vi "ModelSimulationAdv.vi"() -> ()   [LabVIEW 2015]
uses:
  Classes/CAlex2/TypeDef/LowerBodyDim.ctl
  Classes/ForceField/TypeDef/FF_Gains.ctl
  Classes/CAlex2/CAlex2.lvclass
  Classes/CAlex2-Display/CAlex2_Display.lvclass
  Classes/ForceField/ForceField.lvclass
  <vilib>/Platform/TimedLoop/XDataNode/timing_clust.ctl
  <vilib>/Platform/TimedLoop/XDataNode/nitl_modes.ctl
  <vilib>/Platform/TimedLoop/XDataNode/wakeup.ctl
  Classes/ForceField/FF_SetGains.vi
  <vilib>/Analysis/BLAS.llb/dgemv - General Matrix-Vector Product (DBL).vi
  <vilib>/Platform/TimedLoop/XDataNode/XDataNode.xnode
  <vilib>/Platform/TimedLoop/XDataNode/XDNodeRunTimeDep.lvlib
  Classes/SerialChain-Cable/SerialChain-Cable.lvclass
  <vilib>/Analysis/NI_AALBLAS.lvlib
  <vilib>/ptbypt/NI_PtbyPt.lvlib
panel:
  in  "ExtraWeight(kg)":cluster{"Thigh":dbl, "Shank":dbl}
  out "Array":dbl[](array[numeric])
  out "AverageTraj":dbl[][](array[numeric])
  out "Joint Angles 3":dbl(graph)
  out "Ankle Location":T1(graph)
  in  "ForceField":enum16{"Old", "Adv"}(ring)
  out "size(s)":i32[](array[numeric])
  in  "stop":bool
  in  "Speed":dbl(slide) scale=0.1..1.0
  out "Iteration Duration":i64
  out "Joint Angles":T2(graph)
  in  "Reset":bool
  in  "Play":bool
  out "Joint Angles":dbl[][](graph)
  out "AnkleTraj dup":dbl[][](array[numeric])=[[0.37183265375099783, -0.7753745975904054, 0.0], [0.37289482382685957, -0.7748969789550374, 0.0], [0.373493623426573, -0.774628944735343, 0.0], [0.37411977937897245, -0.7743495847216937, 0.0], [0.37433541633017775, -0.7742546779467274, 0.0], [0.37425855125757534, -0.7742906050038265, 0.0], [0.37384605819479033, -0.774472841116272, 0.0], [0.37296121505608076, -0.7748580324475733, 0.0], [0.37170692962948126, -0.7753928087899727, 0.0], [0.3700602785380804, -0.7760822332687248, 0.0], [0.36809143852899284, -0.7768866046659747, 0.0], [0.36568836065849897, -0.7778423221117037, 0.0], [0.36313552913237124, -0.7788278813089, 0.0], [0.3601118692047611, -0.7799584423849573, 0.0], [0.3572321518028252, -0.7809989203616594, 0.0], [0.35378972494099115, -0.7822011715240718, 0.0], [0.35059287638745984, -0.7832774768890238, 0.0], [0.3467578061484453, -0.7845221886070235, 0.0], [0.3432982823348635, -0.7856008298535131, 0.0], [0.33934836631794885, -0.7867910445374475, 0.0], [0.33541324452244614, -0.7879258693076385, 0.0], [0.3314474700295142, -0.789029178751681, 0.0], [0.32715884390484884, -0.7901684748000672, 0.0], [0.3231117563662566, -0.7912012543919054, 0.0], [0.3184724786883741, -0.7923291759292822, 0.0], [0.314162029124302, -0.7933285258974756, 0.0], [0.3094336910282637, -0.7943728574273302, 0.0], [0.3048815845425384, -0.7953276067807286, 0.0], [0.30006249829487697, -0.7962839160327793, 0.0], [0.2952110578635034, -0.797190712968026, 0.0], [0.2903579578045672, -0.7980471058277165, 0.0], [0.2853196096836144, -0.7988732306589323, 0.0], [0.28033113007614985, -0.7996408813366376, 0.0], [0.2749999968937097, -0.8003945622659994, 0.0], [0.27005660632103534, -0.801037842898324, 0.0], [0.26454255052510184, -0.8016912636825307, 0.0], [0.2594436259092606, -0.8022365009693144, 0.0], [0.25384070753157423, -0.8027682840071089, 0.0], [0.24872618036880667, -0.8031916470946026, 0.0], [0.2431628291886645, -0.8035855761699472, 0.0], [0.237850957225839, -0.8038946687980629, 0.0], [0.23220014909346698, -0.8041535831823374, 0.0], [0.22702101700957686, -0.8043243026289639, 0.0], [0.22132859036727104, -0.8044455086499704, 0.0], [0.2161303736065503, -0.8044862796442338, 0.0], [0.21053389057023572, -0.8044652948207722, 0.0], [0.20494606247739322, -0.8043670725575002, 0.0], [0.1996795642462802, -0.804209365734722, 0.0], [0.19387414206660697, -0.803959487604845, 0.0], [0.18860569655152407, -0.8036662143242687, 0.0], [0.18290985424210632, -0.8032746472778416, 0.0], [0.17763852673112943, -0.80284451181639, 0.0], [0.1720637346201731, -0.8023168832402672, 0.0], [0.16670541014624216, -0.8017411231307242, 0.0], [0.16124688034804877, -0.8010855122017577, 0.0], [0.1559100209598843, -0.800376945216661, 0.0], [0.15027133848749125, -0.7995524032540577, 0.0], [0.14506338428592272, -0.7987270788629399, 0.0], [0.13937552048376003, -0.797759709715296, 0.0], [0.134221407365669, -0.7968187612931736, 0.0], [0.12856350148196946, -0.7957309833621973, 0.0], [0.12328836974914918, -0.7946723721393905, 0.0], [0.11749057966524709, -0.7934558221054675, 0.0], [0.11228354529372929, -0.79232840321483, 0.0], [0.10644084465997686, -0.7910119517196016, 0.0], [0.10095291735243607, -0.7897521646217016, 0.0], [0.0949742465260796, -0.7883287460106716, 0.0], [0.08932119053218368, -0.7869521967616934, 0.0], [0.08343964132641435, -0.785483040113578, 0.0], [0.07762692966656667, -0.7839991497744392, 0.0], [0.07135683936790438, -0.7823613070633205, 0.0], [0.0656352421659741, -0.7808325842640069, 0.0], [0.05928812168117539, -0.7791024245187889, 0.0], [0.05326784691840181, -0.7774341704120975, 0.0], [0.04720152296919525, -0.7757070205082308, 0.0], [0.04113274195842884, -0.7739569091825252, 0.0], [0.035073495589465875, -0.7721639239188988, 0.0], [0.029092778510038497, -0.7703645301795483, 0.0], [0.023148090702767327, -0.7685386619074226, 0.0], [0.01733760024588965, -0.7667249115039706, 0.0], [0.011116829949580742, -0.7647479503952259, 0.0], [0.005295634045588998, -0.7628511751120268, 0.0], [-0.00043876377786242204, -0.7609635946087108, 0.0], [-0.006342201549036891, -0.7589715759608368, 0.0], [-0.011929098616239558, -0.7570671623466152, 0.0], [-0.01774704906579269, -0.7550426162385022, 0.0], [-0.023541544919570417, -0.7530086819325862, 0.0], [-0.028957258939425468, -0.7510705734835252, 0.0], [-0.034698138313621396, -0.7490009106985951, 0.0], [-0.04008729757012036, -0.7470392767080659, 0.0], [-0.04574900793341244, -0.7449658783801192, 0.0], [-0.051320828424748444, -0.7429059583063504, 0.0], [-0.05677467622680521, -0.7408648077406232, 0.0], [-0.06226454675363144, -0.7388113211597775, 0.0], [-0.0676389204429593, -0.7367811542598004, 0.0], [-0.0728442278462823, -0.7348053465420634, 0.0], [-0.0782357241582145, -0.7327620142872742, 0.0], [-0.0836394929256932, -0.7306888915502054, 0.0], [-0.0887720530740976, -0.7287105862736893, 0.0], [-0.09389454917760404, -0.726732998735621, 0.0], [-0.09886685610474269, -0.7247987455299281, 0.0], [-0.10383869318508343, -0.722867469607505, 0.0], [-0.10852151332262627, -0.7210522484792419, 0.0], [-0.113409207857913, -0.7191438167829669, 0.0], [-0.11793809256479892, -0.7173929476150898, 0.0], [-0.12254124998410773, -0.7155942737218733, 0.0], [-0.12693686993795159, -0.7139135811901516, 0.0], [-0.13161630521760578, -0.7121241599601726, 0.0], [-0.13581258018488523, -0.7105322342176328, 0.0], [-0.14027599616508363, -0.708881590455069, 0.0], [-0.14450030181936724, -0.7073181803603608, 0.0], [-0.14877060013956167, -0.7057871374866982, 0.0], [-0.1529901004972806, -0.7042851345154005, 0.0], [-0.15718019582987636, -0.7028327254328446, 0.0], [-0.16122244521688234, -0.7014823298049171, 0.0], [-0.1653162445977395, -0.7001418829804374, 0.0], [-0.16929374726325766, -0.69889983696989, 0.0], [-0.1734783601455121, -0.6976299042507634, 0.0], [-0.1770966735528886, -0.6965984300714734, 0.0], [-0.18114059602104032, -0.6955090442952979, 0.0], [-0.184935925009572, -0.6945583547855383, 0.0], [-0.18878423624534665, -0.6937178759316448, 0.0], [-0.19242257225482037, -0.6929866662389191, 0.0], [-0.19615973677621426, -0.6923787119922514, 0.0], [-0.19978175605815884, -0.6919052431255679, 0.0], [-0.20337246600553527, -0.6915188855358476, 0.0], [-0.20682426326370662, -0.6913009470371396, 0.0], [-0.2102769928693155, -0.6912104861499663, 0.0], [-0.2136766885217551, -0.6912634393978416, 0.0], [-0.21702450391347713, -0.6914592765636891, 0.0], [-0.22023476858846222, -0.6917523077549168, 0.0], [-0.22331956369937084, -0.6922362445610458, 0.0], [-0.22636686575938247, -0.6928341134395831, 0.0], [-0.22922823266369957, -0.693665641519721, 0.0], [-0.23192753904420305, -0.6945320687978396, 0.0], [-0.23441321506243118, -0.6956651784863382, 0.0], [-0.2368821322965693, -0.696925825030893, 0.0], [-0.2389547948215033, -0.6982781184291174, 0.0], [-0.24110089510899507, -0.6998876962445497, 0.0], [-0.24287465696440025, -0.7014423387913367, 0.0], [-0.2446742043707928, -0.7033559882647625, 0.0], [-0.24620697206049796, -0.7051112811196629, 0.0], [-0.24764820933713433, -0.7071011257159412, 0.0], [-0.2490230174457068, -0.7091334575948564, 0.0], [-0.25031144941568106, -0.7112798262977702, 0.0], [-0.2514427644386446, -0.7134317431304611, 0.0], [-0.2524929750018052, -0.7155589393861124, 0.0], [-0.25350072515651867, -0.7178246947777653, 0.0], [-0.254380221322995, -0.719927018561745, 0.0], [-0.2552616792998671, -0.722267545511442, 0.0], [-0.2560251567346829, -0.7243835323272311, 0.0], [-0.25680867032020616, -0.726693828115996, 0.0], [-0.2575062201163926, -0.7288676957769442, 0.0], [-0.25816974272182763, -0.7310791287719528, 0.0], [-0.2588252699568618, -0.7333147576395038, 0.0], [-0.25942071073535394, -0.7354274902405354, 0.0], [-0.26003385044795635, -0.7376236111250145, 0.0], [-0.26059715988663323, -0.7396714097897619, 0.0], [-0.2612200470159218, -0.7418991707604716, 0.0], [-0.2617377263415781, -0.7437515197313708, 0.0], [-0.2623744155157041, -0.7459309017913354, 0.0], [-0.26297860529215933, -0.7479575530548156, 0.0], [-0.26358132537438494, -0.7499323028969112, 0.0], [-0.26418697767727833, -0.7518509648059314, 0.0], [-0.264777188672622, -0.7536804383160631, 0.0], [-0.2654198112780903, -0.7556471666562012, 0.0], [-0.2660113415426726, -0.7574533877863839, 0.0], [-0.26659672532042766, -0.7592299713856276, 0.0], [-0.26721269508289713, -0.7611377923270144, 0.0], [-0.2677374078136171, -0.7627913062390148, 0.0], [-0.2683173793927711, -0.7646159197743312, 0.0], [-0.2688101626362109, -0.7661970294615574, 0.0], [-0.26934819761677037, -0.7679265486285046, 0.0], [-0.26984717901082056, -0.7695254496619343, 0.0], [-0.2703347490737253, -0.7711106818083092, 0.0], [-0.27080781288628913, -0.772685255158352, 0.0], [-0.2712845477065148, -0.7742376677421277, 0.0], [-0.27172652145721626, -0.7757296853818727, 0.0], [-0.2721619027572711, -0.7772206684253814, 0.0], [-0.2725457806411501, -0.7786164445559429, 0.0], [-0.27292845491681295, -0.7800794437434274, 0.0], [-0.27325630885853164, -0.7814606263774184, 0.0], [-0.27356303285043426, -0.7828369241522507, 0.0], [-0.2738096548030798, -0.7841627795610804, 0.0], [-0.27402878883574844, -0.7854881888275353, 0.0], [-0.274186228925163, -0.7867626824220673, 0.0], [-0.2743073583286294, -0.7880418506185414, 0.0], [-0.27438738928150447, -0.7892385417358527, 0.0], [-0.2744288342261834, -0.7904689488865955, 0.0], [-0.27441035565444816, -0.7916168524596761, 0.0], [-0.2743634125063062, -0.7927596786734321, 0.0], [-0.2742574236518008, -0.7938718639614482, 0.0], [-0.2741374078183783, -0.7949318812614583, 0.0], [-0.27393887109827364, -0.7960858921110872, 0.0], [-0.2737038263626721, -0.7970832634677752, 0.0], [-0.27341166537655365, -0.798171028508889, 0.0], [-0.2730650444966486, -0.7991339477482047, 0.0], [-0.2726347689249194, -0.8001615272613687, 0.0], [-0.2721534360578481, -0.8011109416356981, 0.0], [-0.27152846952377346, -0.8021552451662262, 0.0], [-0.2708770070319027, -0.8030965774960956, 0.0], [-0.2700172155863569, -0.8041445311604927, 0.0], [-0.26913106108347484, -0.805109858166045, 0.0], [-0.2680068487918412, -0.8061885367916513, 0.0], [-0.2668211514937952, -0.8072184001367346, 0.0], [-0.2654878391152534, -0.8082713109319719, 0.0], [-0.2640317937400684, -0.8093315890960024, 0.0], [-0.26237379458714477, -0.8104381846073867, 0.0], [-0.26068727382666523, -0.8115060789128818, 0.0], [-0.2587495769707093, -0.8126439793150716, 0.0], [-0.25671166521781325, -0.8137870428806746, 0.0], [-0.2546156310828552, -0.8148983667177427, 0.0], [-0.2522381549641083, -0.8161021500951877, 0.0], [-0.2499761368107293, -0.8171988530971919, 0.0], [-0.2474711463082518, -0.8183702224831575, 0.0], [-0.2450060689856413, -0.8194795582043639, 0.0], [-0.24244470949827496, -0.8205997730249799, 0.0], [-0.23993477307897781, -0.821661641193336, 0.0], [-0.2373917701683875, -0.8227104193851609, 0.0], [-0.23480473958874443, -0.8237435592023392, 0.0], [-0.23221757387585168, -0.8247537872359236, 0.0], [-0.22965895358119026, -0.8257246471199526, 0.0], [-0.22711604521835227, -0.8266670541451011, 0.0], [-0.22467194478881602, -0.8275515105824701, 0.0], [-0.2222209361099186, -0.828418398645937, 0.0], [-0.21975095200379302, -0.8292715405676382, 0.0], [-0.21740179408864782, -0.8300646562631699, 0.0], [-0.2150218549152477, -0.8308488450960334, 0.0], [-0.21269276783515087, -0.8316005563577531, 0.0], [-0.2105430277629809, -0.8322800833587969, 0.0], [-0.20827546261146768, -0.8329810666985676, 0.0], [-0.20616611188279502, -0.8336227899995121, 0.0], [-0.20411247571039182, -0.8342342912086944, 0.0], [-0.2019978531568194, -0.8348527927379376, 0.0], [-0.20015106125248622, -0.835383430255904, 0.0], [-0.19815292207435609, -0.8359473626823527, 0.0], [-0.19645607999172088, -0.8364189829271711, 0.0], [-0.19464053492952343, -0.8369158132866583, 0.0], [-0.19307405926458887, -0.837338306633453, 0.0], [-0.19139803881526166, -0.8377833938319692, 0.0], [-0.18962018754632556, -0.8382482281998148, 0.0], [-0.18824260076912852, -0.8386033398660642, 0.0], [-0.1867633360321964, -0.8389793558486134, 0.0], [-0.18547833013150733, -0.8393014955259506, 0.0], [-0.18404141743744645, -0.8396562208809251, 0.0], [-0.18278247041905893, -0.8399627646858725, 0.0], [-0.18140807652754443, -0.8402927271900011, 0.0], [-0.18012494884891897, -0.8405961811142164, 0.0], [-0.1788289309698709, -0.8408988399639594, 0.0], [-0.17747462776908626, -0.8412099050582688, 0.0], [-0.17619382108109571, -0.8415005768042629, 0.0], [-0.17481346130734696, -0.8418093850591277, 0.0], [-0.17340829015016793, -0.8421196068543741, 0.0], [-0.1719694132738892, -0.842432616487675, 0.0], [-0.17047884539720298, -0.8427527384267661, 0.0], [-0.16896770404045502, -0.843072807600878, 0.0], [-0.1673780501531782, -0.84340478181457, 0.0], [-0.16571906452660776, -0.8437464035465461, 0.0], [-0.16404147499149918, -0.8440869618649394, 0.0], [-0.16228213634532412, -0.8444392151349265, 0.0], [-0.16047364442066228, -0.8447957743706607, 0.0], [-0.1586514507170836, -0.8451499896818444, 0.0], [-0.15677822979604894, -0.8455086788850721, 0.0], [-0.15483004182304438, -0.8458762665312334, 0.0], [-0.15283113439288662, -0.8462475387577932, 0.0], [-0.15072388689399357, -0.8466328389003069, 0.0], [-0.14872295822956122, -0.8469927691964696, 0.0], [-0.14650702271158547, -0.847385139741527, 0.0], [-0.14442166132674084, -0.8477481694081889, 0.0], [-0.1422666720786283, -0.8481172868947848, 0.0], [-0.14004673814526042, -0.8484910648578541, 0.0], [-0.13796406790621085, -0.8488358398219539, 0.0], [-0.13572869301500584, -0.8491996022657746, 0.0], [-0.13358391000669767, -0.8495425544447857, 0.0], [-0.13140858934261096, -0.8498843882979255, 0.0], [-0.12928110336475632, -0.8502129140790096, 0.0], [-0.12704531611413403, -0.8505519396803537, 0.0], [-0.12499877452630204, -0.8508567808565243, 0.0], [-0.12287895472414473, -0.8511669920612306, 0.0], [-0.1209871435845552, -0.8514391483290421, 0.0], [-0.11891710432316879, -0.8517318300467451, 0.0], [-0.11706935003037391, -0.8519886162558002, 0.0], [-0.11522229341616635, -0.8522411020733642, 0.0], [-0.11351709372269617, -0.8524704787231319, 0.0], [-0.11174322345590623, -0.8527053249622711, 0.0], [-0.11013622737131207, -0.8529147618458993, 0.0], [-0.10840840557341808, -0.8531364414159233, 0.0], [-0.10701529650561606, -0.8533125360256351, 0.0], [-0.10536501640381091, -0.8535181014042106, 0.0], [-0.10383529190748454, -0.8537057161586962, 0.0], [-0.10238143017378959, -0.8538814096088274, 0.0], [-0.10082932866972373, -0.854066181686951, 0.0], [-0.09936778885974791, -0.8542375272359429, 0.0], [-0.09782548082175646, -0.8544155765474297, 0.0], [-0.0963157931390409, -0.8545871110310665, 0.0], [-0.09474769022157203, -0.854762396513045, 0.0], [-0.09318198152710554, -0.8549345022846709, 0.0], [-0.09154856137331283, -0.8551109351178154, 0.0], [-0.08990834228076758, -0.8552849215694632, 0.0], [-0.088198444687737, -0.8554628953887149, 0.0], [-0.08648663207162453, -0.8556376015115305, 0.0], [-0.08468618696227526, -0.8558175989984749, 0.0], [-0.08287167596264519, -0.8559951191779169, 0.0], [-0.08097949268135497, -0.8561760880823152, 0.0], [-0.07903148956315978, -0.8563579629636042, 0.0], [-0.07704161240048532, -0.8565391221986036, 0.0], [-0.07502566632690028, -0.8567178812545901, 0.0], [-0.07282142574034856, -0.8569078409138489, 0.0], [-0.07076608151912692, -0.8570798219419018, 0.0], [-0.06835711622559534, -0.8572750411585485, 0.0], [-0.06613254008617091, -0.8574492739066633, 0.0], [-0.06355061805798805, -0.8576441765080185, 0.0], [-0.06106420248426459, -0.8578244406207083, 0.0], [-0.05850268624516532, -0.8580025935368184, 0.0], [-0.055736260696897, -0.8581862830569933, 0.0], [-0.05305406859854181, -0.8583558796759434, 0.0], [-0.050262421932745986, -0.8585233303202323, 0.0], [-0.04736702971716894, -0.8586874080081011, 0.0], [-0.044370286732769645, -0.8588467922743324, 0.0], [-0.041531306378691873, -0.858988078838129, 0.0], [-0.03839991406525789, -0.8591328669596852, 0.0], [-0.03510860090786879, -0.8592725569099622, 0.0], [-0.03210990117282504, -0.8593887569585896, 0.0], [-0.028899478532724704, -0.8595012427721156, 0.0], [-0.025823678520056043, -0.8595976180772692, 0.0], [-0.022617832756158897, -0.859685893536088, 0.0], [-0.01946792858750787, -0.8597607865717275, 0.0], [-0.016388976031073983, -0.8598223381851606, 0.0], [-0.013167726108472215, -0.8598744713081619, 0.0], [-0.010251216509382356, -0.8599107816034928, 0.0], [-0.007019606669465612, -0.8599386941101604, 0.0], [-0.004153763070109593, -0.8599528219186598, 0.0], [-0.0010910884263649967, -0.859956271256102, 0.0], [0.001778124897785133, -0.8599488154199191, 0.0], [0.004647360708474891, -0.8599306751781897, 0.0], [0.007474672404238891, -0.8599024106472315, 0.0], [0.010355664289539997, -0.8598628527522061, 0.0], [0.013069752444236783, -0.8598149395701302, 0.0], [0.01565097819637608, -0.8597608617255861, 0.0], [0.018464189530154194, -0.8596909628742213, 0.0], [0.020971142300671836, -0.8596199682875074, 0.0], [0.02373313451673249, -0.8595314661119279, 0.0], [0.026241847162740032, -0.859442077835348, 0.0], [0.02896355621561992, -0.8593351658357784, 0.0], [0.031561304479187265, -0.8592236525940238, 0.0], [0.03421311230968467, -0.8591002220711204, 0.0], [0.03692509235563076, -0.8589642546371237, 0.0], [0.03966199276671022, -0.8588161876750965, 0.0], [0.04233321473653107, -0.8586615454189499, 0.0], [0.04500898398863215, -0.8584958883725464, 0.0], [0.04774489004844869, -0.8583155343357147, 0.0], [0.05036852727515613, -0.8581319745907592, 0.0], [0.05317339321487827, -0.8579249192964813, 0.0], [0.055798644180901726, -0.8577203942779614, 0.0], [0.05851843148614406, -0.8574972766947069, 0.0], [0.06122614212627327, -0.8572652071642932, 0.0], [0.0640107179210352, -0.8570141205377868, 0.0], [0.066691883462811, -0.8567630906049144, 0.0], [0.06954690889383948, -0.8564847261034455, 0.0], [0.07222822506589574, -0.8562138180184402, 0.0], [0.07542250396384256, -0.8558816792851693, 0.0], [0.0781719810318635, -0.8555841106898108, 0.0], [0.08139890251569763, -0.8552270930677746, 0.0], [0.08450389791313062, -0.8548725915629658, 0.0], [0.08773326273118319, -0.8544901441486166, 0.0], [0.09090642645414464, -0.854104783508446, 0.0], [0.09423999387967696, -0.8536883980846051, 0.0], [0.09750187723856218, -0.8532660006092561, 0.0], [0.1009018177825952, -0.8528153371744314, 0.0], [0.1041666709264735, -0.8523687507035258, 0.0], [0.10761630667780497, -0.8518868915180231, 0.0], [0.11074845594993368, -0.8514315701081683, 0.0], [0.11421463157333586, -0.8509189161811136, 0.0], [0.11738828663298527, -0.8504348099207938, 0.0], [0.12061003539211371, -0.8499339763267597, 0.0], [0.12377847214797102, -0.8494281235205758, 0.0], [0.12708458841920295, -0.8488895628043887, 0.0], [0.13016688827131792, -0.848375207862568, 0.0], [0.1333610916696111, -0.8478330249247403, 0.0], [0.13647626865151896, -0.8472928272446203, 0.0], [0.1396480343049928, -0.8467332182857404, 0.0], [0.14274536276537236, -0.8461742791491627, 0.0], [0.14598771932507743, -0.845581902804462, 0.0], [0.14890986227024136, -0.8450377521723433, 0.0], [0.1522270134213003, -0.8444105384630858, 0.0], [0.15532553945701422, -0.8438148464185712, 0.0], [0.15845498938830296, -0.8432043069254598, 0.0], [0.1614889015454986, -0.8426028519161191, 0.0], [0.1645666116878986, -0.841982843672705, 0.0], [0.1675741369540738, -0.8413686429892312, 0.0], [0.17046967399268204, -0.8407689299249975, 0.0], [0.17340469189720858, -0.8401536828041312, 0.0], [0.17612716517541172, -0.8395760151571943, 0.0], [0.17892301069413136, -0.8389753104777607, 0.0], [0.18165778429941154, -0.838381186768423, 0.0], [0.18415151787095663, -0.8378335332382447, 0.0], [0.18669339618022673, -0.8372717339545527, 0.0], [0.18905363464157615, -0.8367432081061068, 0.0], [0.19135324597196007, -0.8362278102306224, 0.0], [0.19363888485475977, -0.835709303566087, 0.0], [0.19590158290764315, -0.8351967462825411, 0.0], [0.1981084640038252, -0.8346931100438553, 0.0], [0.20033022729261885, -0.83418524884933, 0.0], [0.20259605689944776, -0.833665550948625, 0.0], [0.204901890440473, -0.8331324000017677, 0.0], [0.2073263385550317, -0.832570336107055, 0.0], [0.20979040241561736, -0.8319946891819853, 0.0], [0.21248896162809622, -0.8313596057342136, 0.0], [0.2150565630550852, -0.830750022361683, 0.0], [0.2179907905266466, -0.8300447061782359, 0.0], [0.22079792544536309, -0.8293630186961082, 0.0], [0.22378446417723674, -0.828627414972503, 0.0], [0.2267101506860001, -0.8278975003771158, 0.0], [0.22993841717261024, -0.8270787890188973, 0.0], [0.23296514070884217, -0.8263008813606285, 0.0], [0.23615343240265585, -0.825468032758038, 0.0], [0.23921892931773792, -0.824654146994607, 0.0], [0.24252743094243195, -0.8237622193619464, 0.0], [0.24557349850440333, -0.822927335774595, 0.0], [0.24877572680170718, -0.8220370922257707, 0.0], [0.2517901425415419, -0.8211837168887886, 0.0], [0.2550128597037762, -0.8202592598352787, 0.0], [0.2578981453454072, -0.8194170964491038, 0.0], [0.2610146145836939, -0.8184957785318425, 0.0], [0.26388548653260374, -0.8176323515222093, 0.0], [0.26675057068370417, -0.8167598230099201, 0.0], [0.2695178402960374, -0.8159053242860688, 0.0], [0.27232531831880064, -0.8150257302621371, 0.0], [0.2749435624610046, -0.8141965433092677, 0.0], [0.27769696793626447, -0.8133118176593679, 0.0], [0.2802063212271111, -0.8124965604428448, 0.0], [0.28285269700734705, -0.8116261291001333, 0.0], [0.2853681052357947, -0.8107887997983884, 0.0], [0.2879112490380726, -0.8099321466933329, 0.0], [0.29039526587283787, -0.8090850305927854, 0.0], [0.29276494026480815, -0.8082681838187457, 0.0], [0.2952725006554657, -0.8073934026365, 0.0], [0.29755405702431903, -0.8065889536156597, 0.0], [0.30000649001559, -0.8057148373344248, 0.0], [0.30223738185111115, -0.8049108096460895, 0.0], [0.3046260290344815, -0.8040405201512473, 0.0], [0.3067465864499216, -0.8032598902083721, 0.0], [0.30900254170215785, -0.802421524563772, 0.0], [0.31098481023502517, -0.801677341465603, 0.0], [0.31308613919629935, -0.8008815451475904, 0.0], [0.31489460499025823, -0.8001904675097968, 0.0], [0.31681506677079885, -0.7994505313042297, 0.0], [0.318505013060268, -0.7987939467899835, 0.0], [0.3203037190245617, -0.7980890086554995, 0.0], [0.3219528440359778, -0.797437071431937, 0.0], [0.32366911018666833, -0.7967521646516664, 0.0], [0.3254216921724232, -0.7960458041553538, 0.0], [0.32712704621727495, -0.795351518173878, 0.0], [0.3290293092012364, -0.7945688036216725, 0.0], [0.3308473666700556, -0.7938127295055969, 0.0], [0.33296376759017093, -0.7929229766820975, 0.0], [0.334932220404212, -0.7920863292322609, 0.0], [0.337180395170873, -0.7911206162524718, 0.0], [0.33935673859080817, -0.7901757239041011, 0.0], [0.34163736031660535, -0.78917503855842, 0.0], [0.34403234844406066, -0.7881136551471178, 0.0], [0.3461839921685177, -0.7871504177049249, 0.0], [0.3486115004743213, -0.7860538836945515, 0.0], [0.35060255233506765, -0.7851460399823808, 0.0], [0.3527788851356809, -0.7841473112638164, 0.0], [0.3545976299933107, -0.783306390513216, 0.0], [0.3564533527366056, -0.7824443739675445, 0.0], [0.35805011929249386, -0.7816995677937202, 0.0], [0.3595694107302563, -0.7809884623637544, 0.0], [0.36091162353209566, -0.7803607510769153, 0.0], [0.36214910788724897, -0.7797817215270448, 0.0], [0.36333794462930863, -0.7792279294893029, 0.0], [0.36447171537128087, -0.778702413584851, 0.0], [0.3654410245748628, -0.7782563066425645, 0.0], [0.36657730897196084, -0.777737299247806, 0.0], [0.36742052655401913, -0.7773538478430514, 0.0], [0.36858563173190617, -0.7768266280103568, 0.0], [0.36942057890451696, -0.7764499087497039, 0.0], [0.37061429689154934, -0.7759115502341369, 0.0], [0.3714117663491737, -0.7755523212160451, 0.0]]
  in  "Relative Weight":dbl[](array[numeric]) format="%#.3f"
  out "ActualTorque":dbl[](array[numeric]) format="%#.6f"
  in  "Gains":T3
  out "FieldForce":dbl[](array[numeric])
  in  "InitDisplay":bool
  out "ActiveTraj":dbl[][](array[numeric])
  in  "BodyWtComp?(F)":bool
  in  "CuffWtComp?(F)":bool=TRUE
  in  "InitFF":bool
  in  "Weight(1e-6)":dbl=1e-06 format="%#_13g"
  in  "LegProperties":T4={"BodyDim(m)"={"ThighLt"=0.42, "ShankLt"=0.42, "HipWd"=0.32}, "BodyWt(kg)"={"Thigh"=0.0, "Shank"=0.0}, "CuffLoc(m)"={"HipCuffWd"=0.4, "HipCuffHt"=0.1, "HipCuffFwdShift"=0.0, "ThighCuffToKnee"=0.25, "ThighCuffDist"=0.04, "ShankCuffToKnee"=0.15}}
  out "FieldForceComp":dbl[](array[numeric]) format="%#.3f"
  out "ClosestPt":dbl[](array[numeric]) format="%#.3f"
  in  "TorqueError":T5
  in  "3D Curve":refnum<k7>(container)
  out "Torque Error":dbl[](array[numeric]) format="%#.3f"
  in  "QuadProg":enum16{"Tight", "Loose", "Adv"}(ring)
  out "Jacobian":dbl[][](array[numeric]) format="%#.4f"
  out "Joint Velocity (rad)":dbl[](array[numeric])
  out "Joint Angles (rad)":dbl[](array[numeric])
  out "DesiredTorque":dbl[](array[numeric]) format="%#.3f"
  in  "Update Arm":bool
  out "Iteration Duration 2":i64
  out "Ankle Position":dbl[](array[numeric]) format="%#.6f"
  out "Solved 2":bool
  out "Planned Tension":dbl[](array[numeric])
  in  "Joint Velocity (deg)":dbl[](array[numeric])=[0.0, 0.0, 0.0, 0.0]
  in  "Leg Joint Angles (deg)":dbl[](array[numeric])=[0.0, 0.0, 0.0, 0.0]
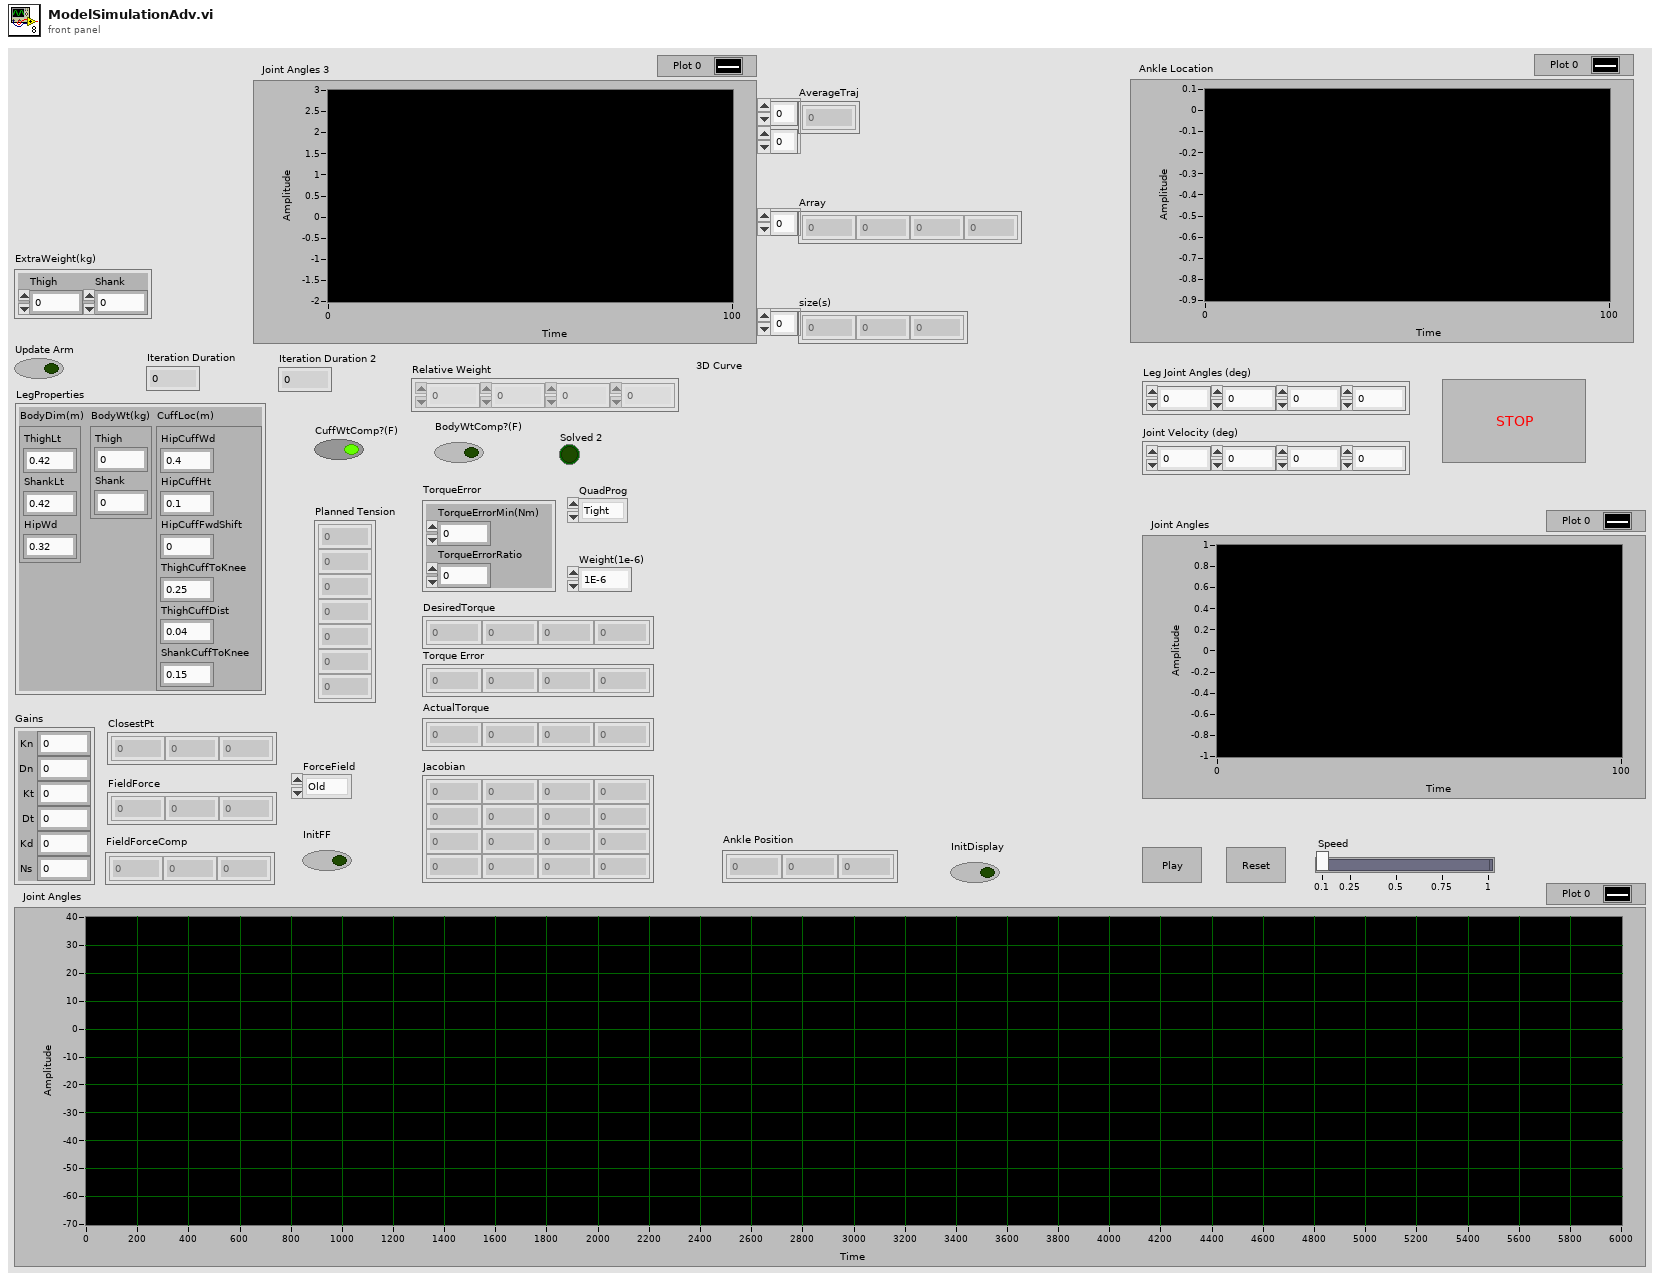
[diagram p1: front panel]
types:
  T1 = cluster{"EndEffInGCS[0]":dbl, "EndEffInGCS[1]":dbl, "EndEffInGCS[2]":dbl}
  T2 = cluster{"Leg Joint Angles (deg)[0]":dbl, "Leg Joint Angles (deg)[1]":dbl, "Leg Joint Angles (deg)[2]":dbl, "Leg Joint Angles (deg)[3]":dbl}
  T3 = typedef "ForceField.lvclass/FF_Gains.ctl" = cluster{"Kn":dbl, "Dn":dbl, "Kt":dbl, "Dt":dbl, "Kd":dbl, "Ns":dbl}
  T4 = typedef "CAlex2.lvclass/LowerBodyDim.ctl" = cluster{"BodyDim(m)":cluster{"ThighLt":dbl, "ShankLt":dbl, "HipWd":dbl}, "BodyWt(kg)":cluster{"Thigh":dbl, "Shank":dbl}, "CuffLoc(m)":cluster{"HipCuffWd":dbl, "HipCuffHt":dbl, "HipCuffFwdShift":dbl, "ThighCuffToKnee":dbl, "ThighCuffDist":dbl, "ShankCuffToKnee":dbl}}
  T5 = cluster{"TorqueErrorMin(Nm)":dbl, "TorqueErrorRatio":dbl}
  T6 = cluster{"Name":string, "Color":u32, "Style":i32, "Point Style":i32, "Name Visible":bool, "Allow Drag":bool, "Annotation Mode":i32, "Plot":i32, "Index":i32, "Position":cluster{"X":dbl, "Y":dbl}, "X Scale":u32, "Y Scale":u32, "Show Arrow":bool, "Lock Name":bool, "Plot Area":i32, "Label Offset":cluster{"X":dbl, "Y":dbl}}
  T7 = typedef "XDNodeRunTimeDep.lvlib/timing_clust.ctl" = cluster{"Expected End [f-1]":u64, "Actual End [f-1]":u64, "Finished Late? [f-1]":bool, "Expected End [i-1]":u64, "Actual End [i-1]":u64, "Finished Late? [i-1]":bool, "Expected Start [i]":u64, "Actual Start [i]":u64, "Expected Start [f]":u64, "Actual Start [f]":u64, "Source Name":string, "Structure Name":string, "Period":i64, "Deadline":i64, "Offset":i64, "Start":i64, "Priority":i32, "Timeout":i32, "Mode":T8, "Wakeup Reason":T9, "Error":errorcluster, "Source Type":string, "Secondary Source Type":string, "Global End Time":u64, "Global Start Time":u64, "Frame Duration":u64, "Iteration Duration":u64, "Assigned CPU":i32, "I/O Scan Engine Mode":u32}
  T8 = typedef "XDNodeRunTimeDep.lvlib/nitl_modes.ctl" = enum32{"No Change", "Process missed periods, maintain original phase", "Discard missed periods, maintain original phase", "Process missed periods, ignore original phase", "Discard missed periods, ignore original phase"}
  T9 = typedef "XDNodeRunTimeDep.lvlib/wakeup.ctl" = enum32{"Normal", "Aborted", "Asynchronous wakeup", "Timing source error", "Timed loop error", "Timeout"}
  T10 = cluster{"AxisLabel":string[], "AxisMax":dbl[], "AxisMin":dbl[]}
  T11 = typedef "SerialChain.lvclass/PointOnBody.ctl" = cluster{"Coord4":dbl[], "ID":i32}
  T12 = typedef "NI_Matrix.lvlib/RealMatrix.ctl" = dbl[][]
  T13 = cluster{"Name":string, "Color":u32, "Style":i32, "Point Style":i32, "Name Visible":bool, "Allow Drag":bool, "Annotation Mode":i32, "Plot":i32, "Index":i32, "Position":cluster{"X":dbl, "Y":dbl}, "X Scale":u32, "Y Scale":u32, "Show Arrow":bool, "Lock Name":bool, "Plot Area":i32, "Label Offset":cluster{"X":dbl, "Y":dbl}}[]
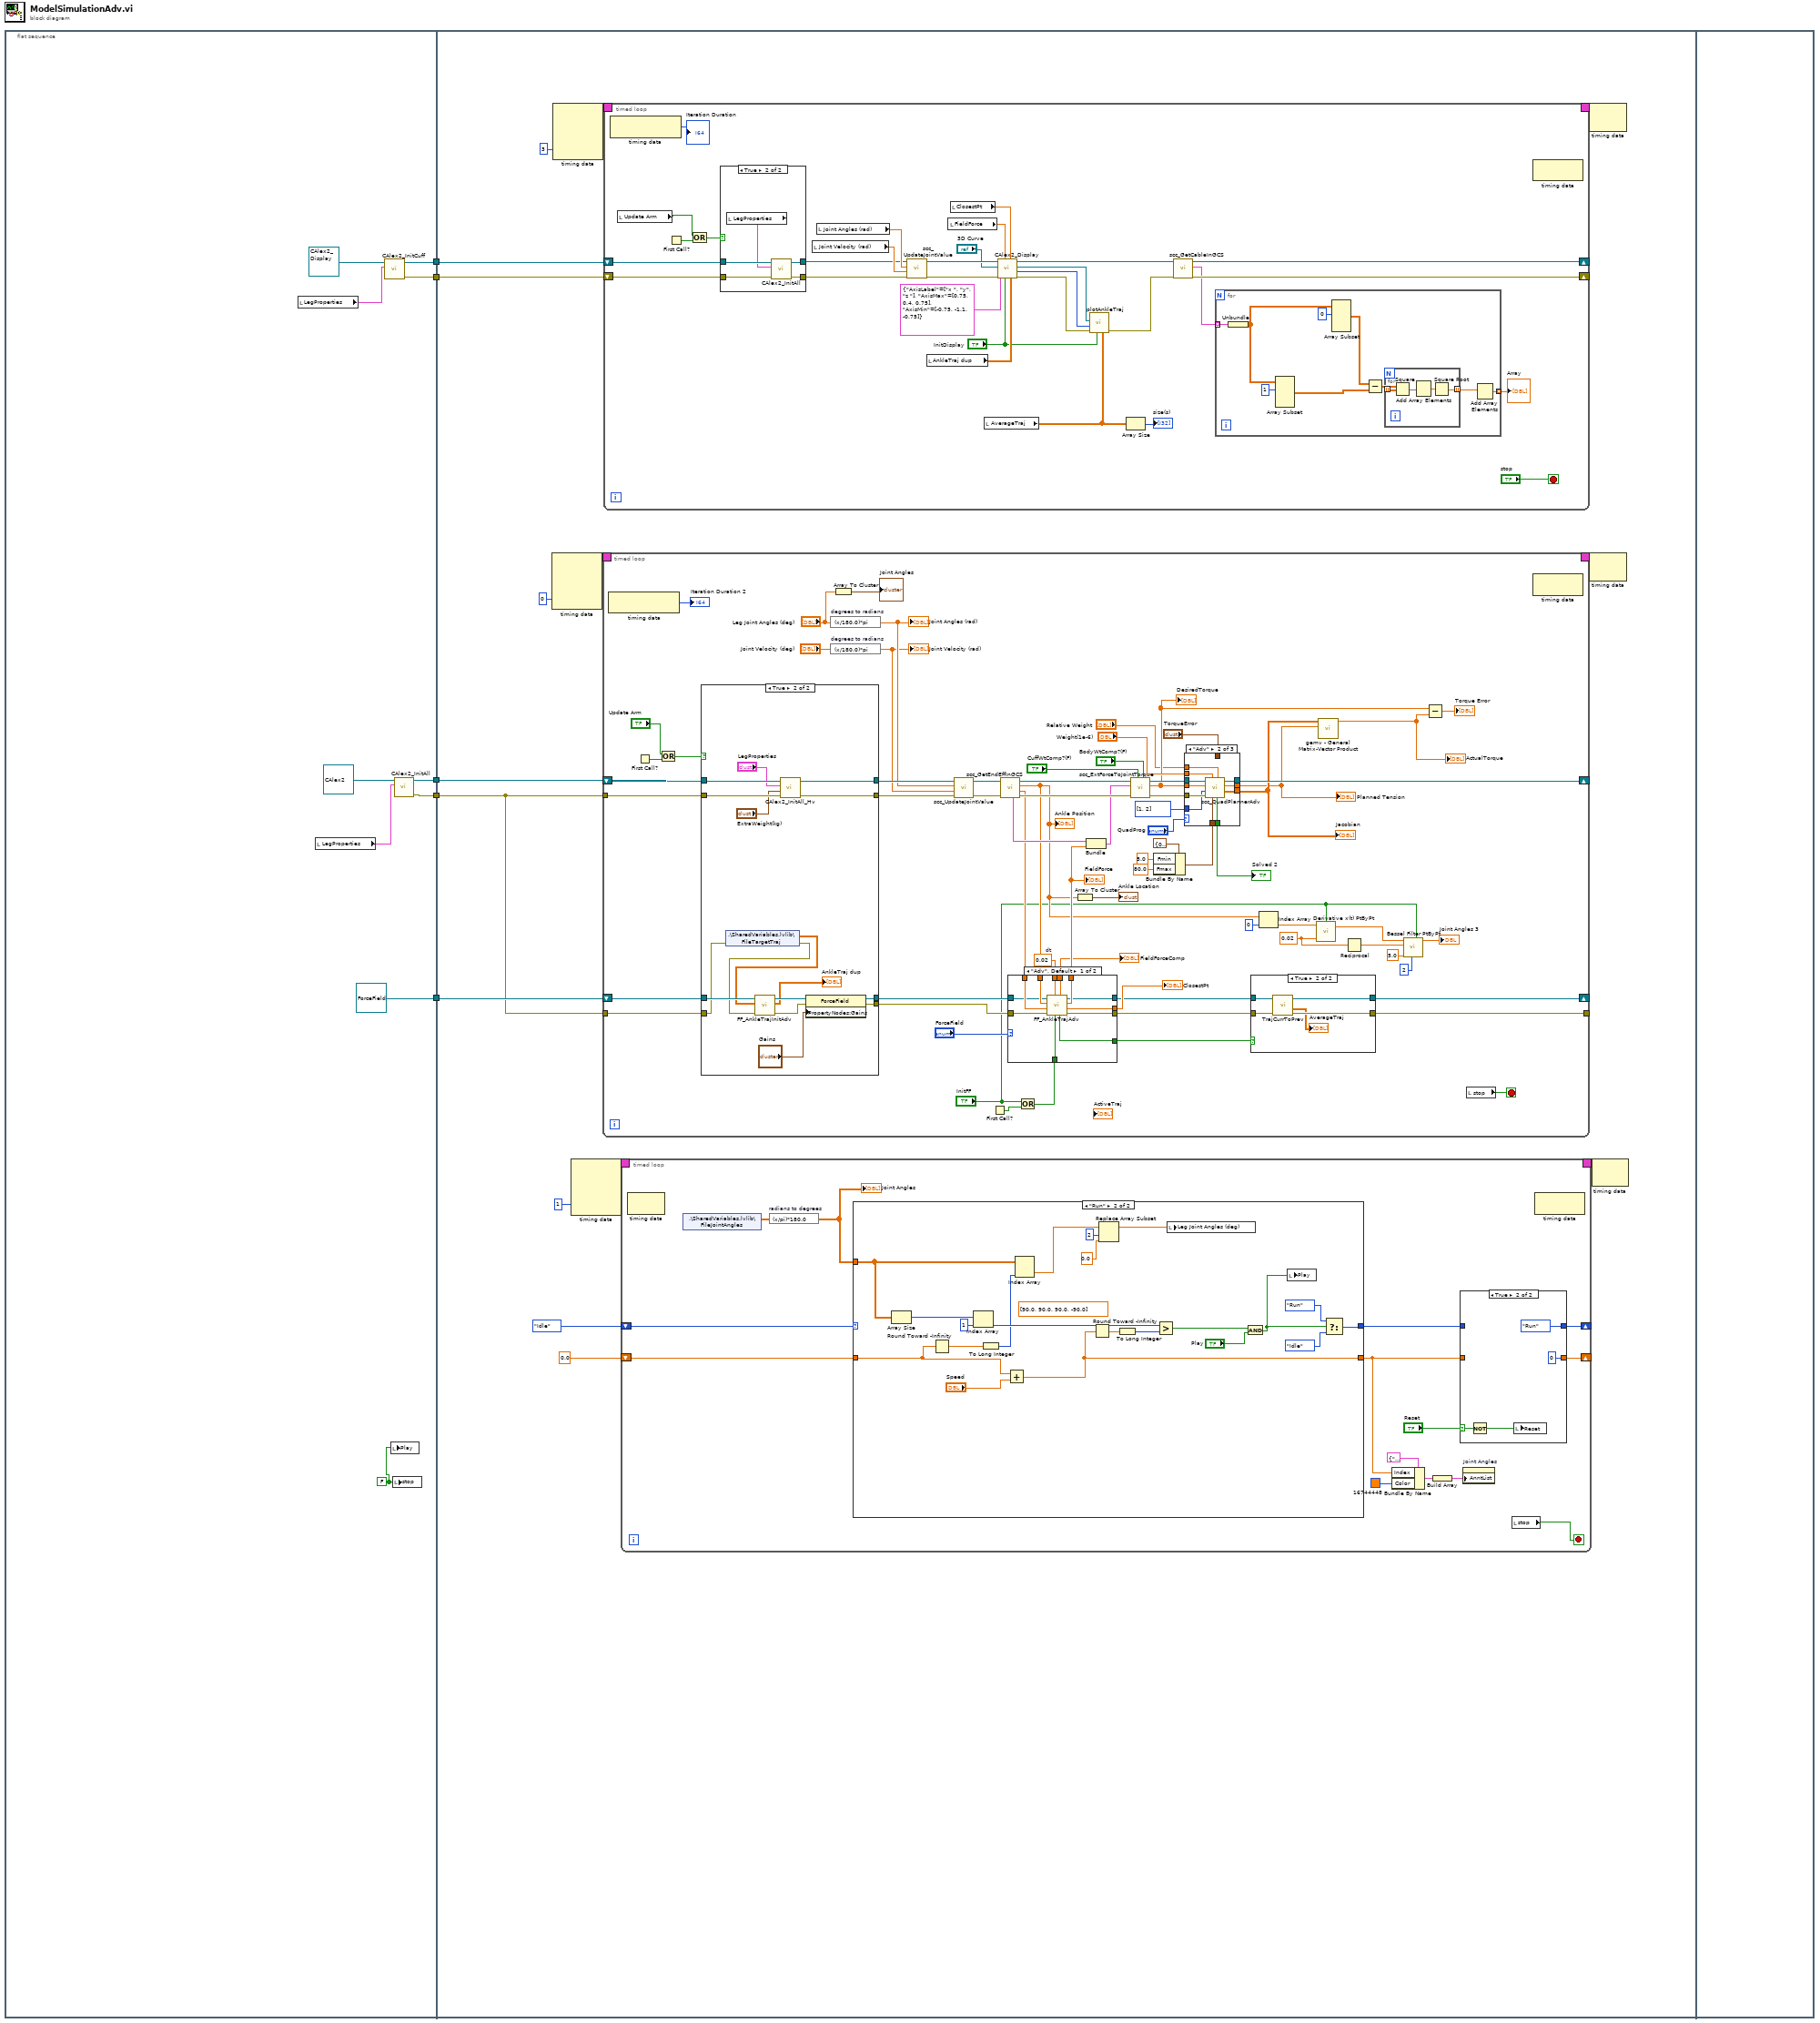
[diagram p0: block diagram]
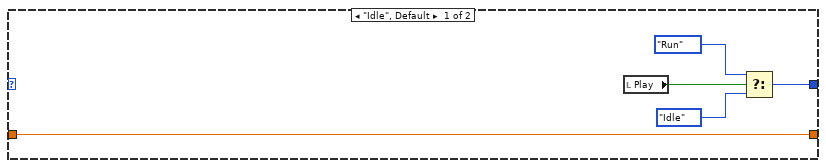
[diagram p3: hidden frame]
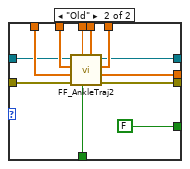
[diagram p5: hidden frame]
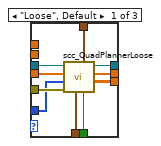
[diagram p7: hidden frame]
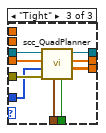
[diagram p8: hidden frame]
diagram:
  n1 = flat-sequence {
    tunnel: [w11] -> w5
    tunnel: [w10] -> w4
    tunnel: [w14] -> w3
    tunnel: [w13] -> w2
    tunnel: [refnum<class "ForceField.lvclass"> refnum ("ForceField")] -> w1
    tunnel: w5 -> [w29]
    tunnel: w4 -> [w21]
    tunnel: w3 -> [w26]
    tunnel: w2 -> [w25]
    tunnel: w1 -> [w22]
    frame #0 {
      w6 = FALSE ("stop")
      n2 = local read "LegProperties"() -> (w7:T4)
      n3 = local read "LegProperties"() -> (w8:T4)
      n4 = call-dynamic "CAlex2_InitCuff.vi"("LegProperty"=w7, "CAlex2 in"=refnum<class "CAlex2_Display.lvclass"> refnum ("CAREX_NYU")) -> ("error out"=w13:errorcluster, "CAlex2 out"=w14:refnum<class "CAlex2_Display.lvclass">)  [unwired: 8 in]
      n5 = local write "Play"(w6) -> ()
      n6 = local write "stop"(w6) -> ()
      n7 = call-dynamic "CAlex2_InitAll.vi"("LegProperties"=w8, "CAlex2 in"=refnum<class "CAlex2.lvclass"> refnum ("CAREX_NYU")) -> ("error out"=w10:errorcluster, "CAlex2 out"=w11:refnum<class "CAlex2.lvclass">)  [unwired: 8 in]
    }
    frame #1 {
      n8 = node-c288(0 ("Processor")) -> (w31:T7)  [unwired: 3 in]
      n9 = node-c288(3 ("Processor")) -> (w28:T7)  [unwired: 3 in]
      n10 = node-c288(1 ("Processor")) -> (w24:T7)  [unwired: 3 in]
      n11 = timed-loop {
        timing: w31 -> [_]
        timing-out: [_] -> w30
        shift-right: [w197] -> _
        shift-left: w29 -> [w196]
        tunnel: w21 -> [w194]
        shift-right: [w167] -> _
        shift-left: w22 -> [w159]
        tunnel: [w165] -> _
        tunnel: w21 -> [w160]
        stop <- w156 stop-if-true
        w144 = 0.02 ("dt")
        w163 = 0.02  # dt
        n12 = node-c288() -> (→"Iteration Duration 2":i64)  [unwired: 1 in]
        n13 = First Call?() -> (First Call?: T/F=w189:bool)
        n14 = Or(x="Update Arm", y=w189) -> (x .or. y?=w191:bool)
        n15 = case shown="True" w191 {
          tunnel: w196 -> [w273 w289]
          tunnel: [w273 w288] -> w195
          tunnel: w194 -> [w272 w285]
          tunnel: [w272 w287] -> w184
          tunnel: [w271 w283] -> w162
          tunnel: [w270 w282] -> w161
          tunnel: w160 -> [w270 w277]
          tunnel: w159 -> [w271 w279]
          frame False {
          }
          frame True {
            n16 = shared-variable ".\\SharedVariables.lvlib\\FileTargetTraj"(error in=w277) -> (w278:dbl[][], error out=w276:errorcluster)
            n17 = call "FF_AnkleTrajInitAdv.vi"("error in (no error)"=w276, "AnkleTraj"=w278, "Force Field Controller in"=w279) -> ("error out"=w280:errorcluster, "AnkleTraj dup"=→"AnkleTraj dup":dbl[][], "Force Field Controller out"=w281:refnum<class "ForceField.lvclass">)  [unwired: 6 in]
            n18 = call-dynamic "CAlex2_InitAll_Hv.vi"("error in (no error)"=w285, "ExtraWeight(kg)"="ExtraWeight(kg)", "LegProperties"="LegProperties", "CAlex2 in"=w289) -> ("error out"=w287:errorcluster, "CAlex2 out"=w288:refnum<class "CAlex2.lvclass">)  [unwired: 6 in]
            n19 = property class="ForceField"(reference=w281, error in=w280, "PropertyNodes:Gains"="Gains") -> (reference out=w283:refnum<class "ForceField.lvclass">, error out=w282:errorcluster)
          }
        }
        n20 = expression code="(x/180.0)*pi" "degrees to radians"("Leg Joint Angles (deg)") -> (w171:dbl[])
        "Joint Angles (rad)" <- w171
        n21 = expression code="(x/180.0)*pi" "degrees to radians"("Joint Velocity (deg)") -> (w170:dbl[])
        "Joint Velocity (rad)" <- w170
        n22 = Array To Cluster(array="Leg Joint Angles (deg)") -> (cluster=→"Joint Angles":T2)
        n23 = call-dynamic "scc_UpdateJointValue.vi"("error in (no error)"=w184, "JointSpeed (rad|m|s)"=w170, "JointValue (rad|m)"=w171, "C-Alex in"=w195) -> ("error out"=w207:errorcluster, "C-Alex out"=w208:refnum<class "CAlex2.lvclass">)  [unwired: 6 in]
        n24 = First Call?() -> (First Call?: T/F=w155:bool)
        n25 = call "scc_GetEndEffInGCS.vi"("error in (no error)"=w207, "SerialChain_Cable in"=w208) -> ("error out"=w183:errorcluster, "EndEffVInGCS"=w180:dbl[], "EndEffInGCS"=w151:dbl[], "SerialChain_Cable out"=w205:refnum<class "CAlex2.lvclass">, "EndEffPos"=w206:T11)  [unwired: 5 in]
        "Ankle Position" <- w151
        n26 = Or(x="InitFF", y=w155) -> (x .or. y?=w154:bool)
        n27 = case shown="\"Adv\", Default" "ForceField" {
          tunnel: w151 -> [w220 w232]
          tunnel: w180 -> [w219 w231]
          tunnel: [w218 w230] -> w179
          tunnel: [w217 w229] -> w176
          tunnel: [w216 w228] -> w175
          tunnel: [w215 w227] -> w168
          tunnel: [w214 w226] -> w166
          tunnel: [w213 FALSE ("UpdateTrajPrev")] -> w164
          tunnel: w163 -> [w212 w225]
          tunnel: w162 -> [w211 w224]
          tunnel: w161 -> [w210 w223]
          tunnel: w154 -> [w209 w221]
          frame "Adv", Default {
            n28 = call "FF_AnkleTrajAdv.vi"("Init"=w209, "dt"=w212, "error in (no error)"=w210, "AnkleVelocity"=w219, "AnkleInGCS"=w220, "Force Field Controller in"=w211) -> ("error out"=w214:errorcluster, "ClosestPoint"=w216:dbl[], "ForceXYZ"=w218:dbl[], "Force Field Controller out"=w215:refnum<class "ForceField.lvclass">, "UpdateTrajPrev"=w213:bool, "ForceNTD"=w217:dbl[])
          }
          frame "Old" {
            n29 = call "FF_AnkleTraj2.vi"("Init"=w221, "dt"=w225, "error in (no error)"=w223, "AnkleVelocity"=w231, "AnkleInGCS"=w232, "Force Field Controller in"=w224) -> ("error out"=w226:errorcluster, "ClosePt"=w228:dbl[], "Force"=w230:dbl[], "Force Field Controller out"=w227:refnum<class "ForceField.lvclass">, "ForceComp"=w229:dbl[])  [unwired: 1 in]
          }
        }
        "ClosestPt" <- w175
        "FieldForceComp" <- w176
        "FieldForce" <- w179
        n30 = Array To Cluster(array=w151) -> (cluster=→"Ankle Location":T1)
        n31 = Bundle("EndEffPos"=w206, "Force"=w179) -> (w178:cluster{"EndEffPos":T11, "Force":dbl[]})  [unwired: 1 in]
        n32 = call "scc_ExtForceToJointTorque.vi"("BodyWtComp?(F)"="BodyWtComp?(F)", "CuffWtComp?(F)"="CuffWtComp?(F)", "error in (no error)"=w183, "External Force (In GCS)"=w178, "SerialChain_Cable in"=w205) -> ("error out"=w204:errorcluster, "DesiredTorque(Nm)"=w174:dbl[], "SerialChain_Cable out"=w203:refnum<class "CAlex2.lvclass">)  [unwired: 4 in]
        "DesiredTorque" <- w174
        n33 = Bundle By Name(cluster=cluster{"Fmin":dbl, "Fmax":dbl} {"Fmin"=0.0, "Fmax"=0.0} ("F range"), "Fmin"=5.0, "Fmax"=80.0) -> (w201:cluster{"Fmin":dbl, "Fmax":dbl})
        n34 = case shown="\"Adv\"" "QuadProg" {
          tunnel: w204 -> [w249 w260 w269]
          tunnel: w203 -> [w248 w259 w268]
          tunnel: w174 -> [w247 w253 w267]
          tunnel: w201 -> [w246 w255 w266]
          tunnel: [w242 w257 w265] -> w186
          tunnel: [w245 w254 w262] -> w198
          tunnel: [w244 w258 w264] -> w197
          tunnel: [w243 w256 w263] -> w187
          tunnel: "TorqueError" -> [w241 _ _]
          tunnel: "Weight(1e-6)" -> [_ w252 _]
          tunnel: "Relative Weight" -> [_ w251 _]
          tunnel: i32[] [1, 2] -> [w240 w250 w261]
          frame "Loose", Default {
            n35 = call "scc_QuadPlannerLoose.vi"("TorqueError(0)"=w241, "F range"=w246, "error in (no error)"=w249, "LockedJoint"=w240, "DesireTorque(Nm)"=w247, "SerialChain_Cable in"=w248) -> ("Jacobian for Cables"=w243:T12, "Planned Tension"=w242:dbl[], "SerialChain_Cable out"=w244:refnum<class "CAlex2.lvclass">, "Solved"=w245:bool)  [unwired: 1 in, 1 out]
          }
          frame "Adv" {
            n36 = call "scc_QuadPlannerAdv.vi"("TorqueRelativeWeight"=w251, "F range"=w255, "Weight(1e-6)"=w252, "error in (no error)"=w260, "LockedJoint(StartFrom0)"=w250, "DesireTorque(Nm)"=w253, "SerialChain_Cable in"=w259) -> ("Jacobian for Cables"=w256:T12, "Planned Tension"=w257:dbl[], "SerialChain_Cable out"=w258:refnum<class "CAlex2.lvclass">, "Solved"=w254:bool)  [unwired: 1 out]
          }
          frame "Tight" {
            n37 = call "scc_QuadPlanner.vi"("F range"=w266, "error in (no error)"=w269, "LockedJoint(StartFrom0)"=w261, "DesireTorque(Nm)"=w267, "SerialChain_Cable in"=w268) -> ("Jacobian for Cables"=w263:T12, "Planned Tension"=w265:dbl[], "SerialChain_Cable out"=w264:refnum<class "CAlex2.lvclass">, "Solved"=w262:bool)  [unwired: 2 in, 1 out]
          }
        }
        "Planned Tension" <- w186
        "Solved 2" <- w198
        "Jacobian" <- w187
        n38 = case shown="True" w164 {
          tunnel: w168 -> [w234 w239]
          tunnel: [w234 w238] -> w167
          tunnel: w166 -> [w233 w237]
          tunnel: [w233 w236] -> w165
          frame False {
          }
          frame True {
            n39 = call "TrajCurrToPrev.vi"("error in (no error)"=w237, "ForceField"=w239) -> ("error out"=w236:errorcluster, "AnkleTraj_array"=→"AverageTraj":dbl[][], "ForceField 2"=w238:refnum<class "ForceField.lvclass">)  [unwired: 6 in, 1 out]
          }
        }
        n40 = Index Array(array=w151, index=0) -> (element=w149:dbl)
        n41 = call <vilib>:"Derivative x(t) PtByPt.vi"("initialize"="InitFF", "dt"=w144, "x"=w149) -> ("dx/dt"=w145:dbl)  [unwired: 1 in, 1 out]
        n42 = call-poly <vilib>:"gemv - General Matrix-Vector Product.vi"("x"=w186, "A"=w187) -> ("dgemv"=w173:dbl[])  [unwired: 8 in, 1 out]
        "ActualTorque" <- w173
        n43 = Reciprocal(x=w144) -> (1/x=w147:dbl)
        n44 = call <vilib>:"Bessel Filter PtByPt.vi"("initialize"="InitFF", "order"=2, "low cutoff freq: fl"=5.0, "sampling freq: fs"=w147, "x"=w145) -> ("Filtered x"=→"Joint Angles 3":dbl)  [unwired: 4 in, 1 out]
        n45 = Subtract(x=w174, y=w173) -> (x-y=→"Torque Error":dbl[])
        n46 = local read "stop"() -> (w156:bool)
        n47 = node-c288() -> ()  [unwired: 1 in, 1 out]
      }
      n48 = timed-loop {
        timing: w28 -> [_]
        timing-out: [_] -> w27
        shift-right: [w87] -> _
        shift-left: w26 -> [w112]
        shift-right: [w86] -> _
        shift-left: w25 -> [w109]
        stop <- "stop" stop-if-true
        n49 = node-c288() -> (→"Iteration Duration":i64)  [unwired: 1 in]
        n50 = local read "Update Arm"() -> (w111:bool)
        n51 = First Call?() -> (First Call?: T/F=w110:bool)
        n52 = Or(x=w111, y=w110) -> (x .or. y?=w113:bool)
        n53 = case shown="True" w113 {
          tunnel: w112 -> [w128 w131]
          tunnel: [w128 w132] -> w106
          tunnel: w109 -> [w127 w130]
          tunnel: [w127 w133] -> w105
          frame False {
          }
          frame True {
            n54 = local read "LegProperties"() -> (w129:T4)
            n55 = call-dynamic "CAlex2_InitAll.vi"("error in (no error)"=w130, "LegProperties"=w129, "CAlex2 in"=w131) -> ("error out"=w133:errorcluster, "CAlex2 out"=w132:refnum<class "CAlex2_Display.lvclass">)  [unwired: 7 in]
          }
        }
        n56 = local read "Joint Velocity (rad)"() -> (w107:dbl[])
        n57 = local read "Joint Angles (rad)"() -> (w108:dbl[])
        n58 = call-dynamic "scc_UpdateJointValue.vi"("error in (no error)"=w105, "JointSpeed (rad|m|s)"=w107, "JointValue (rad|m)"=w108, "C-Alex in"=w106) -> ("error out"=w103:errorcluster, "C-Alex out"=w104:refnum<class "CAlex2_Display.lvclass">)  [unwired: 6 in]
        n59 = local read "AnkleTraj dup"() -> (w98:dbl[][])
        n60 = local read "FieldForce"() -> (w100:dbl[])
        n61 = local read "ClosestPt"() -> (w99:dbl[])
        n62 = local read "AverageTraj"() -> (w90:dbl[][])
        n63 = call "CAlex2_Display.vi"("AnkleTraj"=w98, "ClosePt"=w99, "Init?"="InitDisplay", "Field Force"=w100, "error in (no error)"=w103, "AxisSetting"=T10 {"AxisLabel"=["x ", "y", "z "], "AxisMax"=[0.75, 0.4, 0.75], "AxisMin"=[-0.75, -1.1, -0.75]}, "3D graph in"="3D Curve", "CLX2 in"=w104) -> ("error out"=w93:errorcluster, "LastPlotNum"=w94:i32, "3D graph out"=w95:refnum<k7>, "CLX2 out"=w89:refnum<class "CAlex2_Display.lvclass">)
        n64 = call "plotAnkleTraj.vi"("AnkleTraj"=w90, "Init?"="InitDisplay", "error in (no error)"=w93, "PreviousPlotNum"=w94, "3D graph in"=w95) -> ("error out"=w88:errorcluster)  [unwired: 4 in, 2 out]
        n65 = Array Size(array=w90) -> (size(s)=→"size(s)":i32[])
        n66 = call "scc_GetCableInGCS.vi"("error in (no error)"=w88, "SerialChain_Cable in"=w89) -> ("error out"=w86:errorcluster, "Cables Points"=w85:cluster{"PointInGCS":dbl[][]}[], "SerialChain_Cable out"=w87:refnum<class "CAlex2_Display.lvclass">)  [unwired: 7 in]
        n67 = for {
          tunnel: w85 -> [w122] mode=indexing
          tunnel: [w114] -> w84 mode=indexing
          n68 = Unbundle(w122) -> ("PointInGCS"=w119:dbl[][])
          n69 = Array Subset(array=w119, index (row)=1 ("index")) -> (w117:dbl[][])  [unwired: 3 in]
          n70 = Array Subset(array=w119, index (row)=0 ("index")) -> (w118:dbl[][])  [unwired: 3 in]
          n71 = Subtract(x=w118, y=w117) -> (x-y=w116:dbl[][])
          n72 = for {
            tunnel: w116 -> [w126] mode=indexing
            tunnel: [w123] -> w115 mode=indexing
            n73 = Square(x=w126) -> (x^2=w125:dbl[])
            n74 = Add Array Elements(numeric array=w125) -> (sum=w124:dbl)
            n75 = Square Root(x=w124) -> (sqrt(x)=w123:dbl)
          }
          n76 = Add Array Elements(numeric array=w115) -> (sum=w114:dbl)
        }
        "Array" <- w84
        n77 = node-c288() -> ()  [unwired: 1 in, 1 out]
      }
      n78 = timed-loop {
        timing: w24 -> [_]
        timing-out: [_] -> w23
        shift-right: [w42] -> _
        shift-left: 0.0 -> [w45]
        shift-right: [w34] -> _
        shift-left: enum16{"Idle", "Run"}."Idle" -> [w44]
        stop <- w33 stop-if-true
        n79 = node-c288() -> ()  [unwired: 1 in, 1 out]
        n80 = shared-variable ".\\SharedVariables.lvlib\\FileJointAngles"() -> (w41:dbl[][])  [unwired: 1 in, 1 out]
        n81 = expression code="(x/pi)*180.0" "radians to degrees"(w41) -> (w32:dbl[][])
        "Joint Angles" <- w32
        n82 = case shown="\"Run\"" w44 {
          tunnel: w32 -> [_ w77]
          tunnel: w45 -> [w55 w65]
          tunnel: [w55 w66] -> w39
          tunnel: [w56 w76] -> w35
          frame "Idle", Default {
            n83 = local read "Play"() -> (w54:bool)
            n84 = Select(t=enum16{"Idle", "Run"}."Run", s=w54, f=enum16{"Idle", "Run"}."Idle") -> (s? t:f=w56:enum16{"Idle", "Run"})
          }
          frame "Run" {
            (unwired) dbl[] [90.0, 90.0, 90.0, -90.0] ("AxisMax")
            n85 = Array Size(array=w77) -> (size(s)=w75:i32[])
            n86 = Round Toward -Infinity(1:w65) -> (0:w64:dbl)
            n87 = Index Array(array=w75, index=1) -> (element=w74:i32)
            n88 = To Long Integer(number=w64) -> (32bit integer=w63:i32)
            n89 = Add(x=w65, y="Speed") -> (x+y=w66:dbl)
            n90 = Index Array(array=w77, index (col)=w63) -> (element=w60:dbl[])  [unwired: 1 in]
            n91 = Round Toward -Infinity(1:w66) -> (0:w62:dbl)
            n92 = Replace Array Subset(array=w60, new element=0.0 ("new element/subarray"), index=2) -> (w59:dbl[])
            n93 = To Long Integer(number=w62) -> (32bit integer=w61:i32)
            n94 = Greater?(x=w74, y=w61) -> (0:w72:bool)
            n95 = local write "Leg Joint Angles (deg)"(w59) -> ()
            n96 = And(x=w72, y="Play") -> (x .and. y?=w69:bool)
            n97 = local write "Play"(w69) -> ()
            n98 = Select(t=enum16{"Idle", "Run"}."Run", s=w69, f=enum16{"Idle", "Run"}."Idle") -> (s? t:f=w76:enum16{"Idle", "Run"})
          }
        }
        n99 = Bundle By Name(cluster=T6 {"Name"="", "Color"=0, "Style"=5, "Point Style"=11, "Name Visible"=FALSE, "Allow Drag"=TRUE, "Annotation Mode"=1, "Plot"=0, "Index"=0, "Position"={"X"=0.0, "Y"=0.0}, "X Scale"=0, "Y Scale"=0, "Show Arrow"=FALSE, "Lock Name"=FALSE, "Plot Area"=0, "Label Offset"={"X"=0.0, "Y"=0.0}}, "Index"=w39, "Color"=u32 16744448) -> (w38:T6)
        n100 = Build Array(w38) -> (w37:T13)
        n101 = case shown="True" "Reset" {
          selector: "Reset" -> [_ w50]
          tunnel: w39 -> [w47 _]
          tunnel: [w47 0] -> w42
          tunnel: w35 -> [w46 _]
          tunnel: [w46 enum16{"Idle", "Run"}."Run"] -> w34
          frame False {
          }
          frame True {
            n102 = Not(x=w50) -> (.not. x?=w49:bool)
            n103 = local write "Reset"(w49) -> ()
          }
        }
        n104 = property on="Joint Angles" class="WFGraph (strict)"("AnntList"=w37) -> ()  [unwired: 2 in, 2 out]
        n105 = local read "stop"() -> (w33:bool)
        n106 = node-c288() -> ()  [unwired: 1 in, 1 out]
      }
      n107 = node-c288(w27) -> ()  [unwired: 1 out]
      n108 = node-c288(w30) -> ()  [unwired: 1 out]
      n109 = node-c288(w23) -> ()  [unwired: 1 out]
    }
    frame #2 {
    }
  }
